vi "LINC Handshake.vi"(7 "GUID (optional)":string, 8 "error in (no error)":errorcluster, 11 "LINC session":refnum<class "LINC.lvclass">) -> (0 "error out":errorcluster, 3 "dup LINC session":refnum<class "LINC.lvclass">)   [LabVIEW 2018, in "STEPkgDriver_LINC.lvlib" / "LINC.lvclass"]
uses:
  LINC.lvclass
  LINC Handshake.ctl
  STEPkgDriver_LINC.lvlib
  LINC Command Origin.ctl
  LINC Global Handshake Mode.ctl
  LINC Handshake Internal.ctl
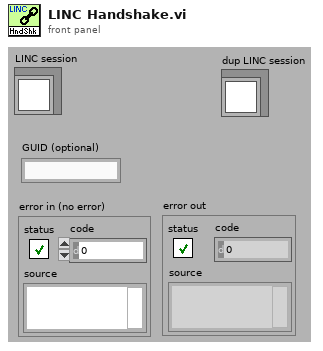
[diagram p1: front panel]
types:
  T1 = typedef "STEPkgDriver_LINC.lvlib/LINC Global Handshake Mode.ctl" = enum16{"INIT", "CLEAR", "ADD_COMMAND", "RMV_COMMAND", "CLR_HANDSHAKE", "SET_HANDSHAKE", "GET_HANDSHAKE"}
  T2 = typedef "STEPkgDriver_LINC.lvlib/LINC Handshake.ctl" = cluster{"ORIGIN":T3, "STATUS":bool, "CODE":i32, "TIME_SECONDS":u32, "TIME_MICROSECONDS":u32, "DATA":string}
  T3 = typedef "STEPkgDriver_LINC.lvlib/LINC Command Origin.ctl" = enum8{"RMT", "LCL"}
  T4 = typedef "STEPkgDriver_LINC.lvlib/LINC Command.ctl" = cluster{"command origin":T3, "command":string, "command data":string}
  T5 = typedef "LVDateTimeRec.ctl" = cluster{"fractional second":dbl, "second":i32, "minute":i32, "hour":i32, "day of month":i32, "month":i32, "year":i32, "day of week":i32, "day of year":i32, "DST":i32}
  T6 = typedef "STEPkgDriver_LINC.lvlib/LINC Handshake Internal.ctl" = cluster{"error":errorcluster, "command data":string}
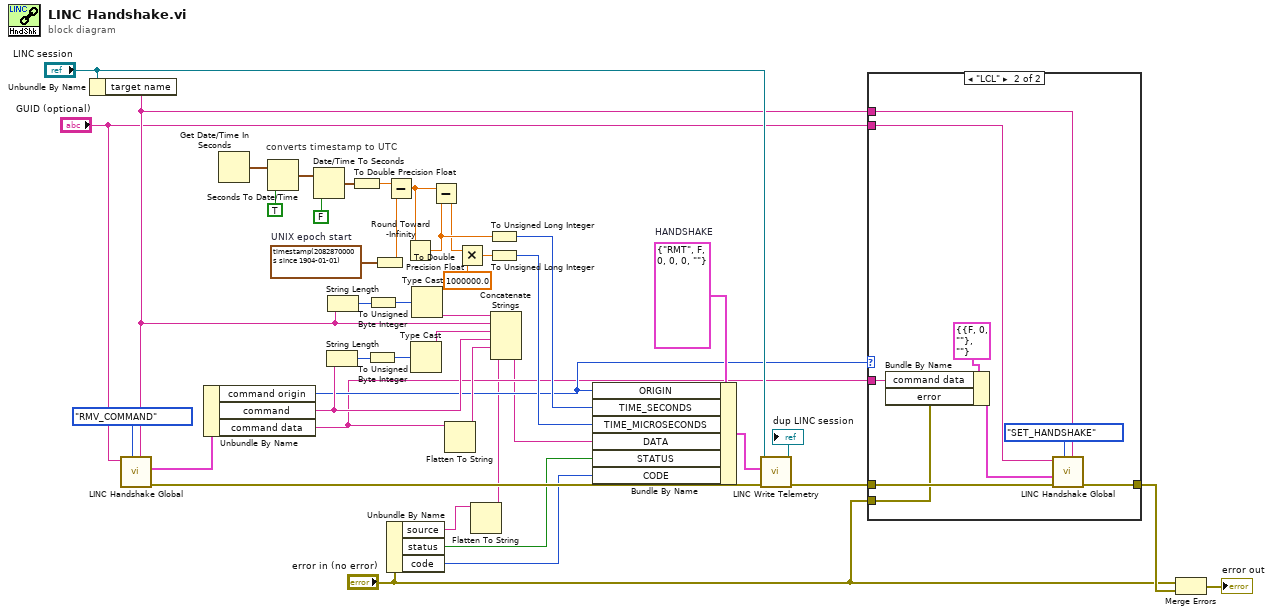
[diagram p0: block diagram]
diagram:
  w29 = timestamp(2082870000 s since 1904-01-01)  # UNIX epoch start
  w32 = T2 {"ORIGIN"=enum."RMT", "STATUS"=FALSE, "CODE"=0, "TIME_SECONDS"=0, "TIME_MICROSECONDS"=0, "DATA"=""}  # HANDSHAKE
  # "converts timestamp to UTC"
  n1 = Unbundle By Name("LINC session") -> ("target name"=w13:string)
  n2 = call "LINC Handshake Global.vi"("target name"=w13, "mode"=LINC_Global_Handshake_Mode."RMV_COMMAND", "GUID"="GUID (optional)") -> ("error out"=w42:errorcluster, "command out"=w9:T4)  [unwired: 5 in, 2 out]
  n3 = Unbundle By Name(w9) -> ("command origin"=w17:T3, "command"=w34:string, "command data"=w7:string)
  n4 = Get Date/Time In Seconds() -> (seconds since 1Jan1904=w8:timestamp)
  n5 = Seconds To Date/Time(time stamp (now)=w8, to UTC (F)=TRUE) -> (date time rec=w19:T5)
  n6 = Date/Time To Seconds(1:FALSE ("is UTC (F)"), 2:w19) -> (0:w18:timestamp)
  n7 = String Length(string=w34) -> (length=w36:i32)
  n8 = String Length(string=w13) -> (length=w40:i32)
  n9 = To Double Precision Float(number=w18) -> (double precision float=w31:dbl)
  n10 = To Unsigned Byte Integer(number=w36) -> (unsigned 8bit integer=w37:u8)
  n11 = To Unsigned Byte Integer(number=w40) -> (unsigned 8bit integer=w39:u8)
  n12 = To Double Precision Float(number=w29) -> (double precision float=w30:dbl)
  n13 = Subtract(x=w31, y=w30) -> (x-y=w28:dbl)
  n14 = Unbundle By Name("error in (no error)") -> ("source"=w3:string, "status"=w5:bool, "code"=w4:i32)
  n15 = Round Toward -Infinity(1:w28) -> (0:w23:dbl)
  n16 = Type Cast(x=w37) -> (*(type *) &x=w35:string)  [unwired: 1 in]
  n17 = Type Cast(x=w39) -> (*(type *) &x=w38:string)  [unwired: 1 in]
  n18 = Subtract(x=w28, y=w23) -> (x-y=w22:dbl)
  n19 = Flatten To String(anything=w7) -> (data string=w33:string)  [unwired: 3 in, 2 out]
  n20 = Multiply(x=w22, y=1000000.0) -> (x*y=w25:dbl)
  n21 = Flatten To String(anything=w3) -> (data string=w2:string)  [unwired: 3 in, 2 out]
  n22 = To Unsigned Long Integer(number=w23) -> (unsigned 32bit integer=w27:u32)
  n23 = To Unsigned Long Integer(number=w25) -> (unsigned 32bit integer=w24:u32)
  n24 = Concatenate Strings(w38, w13, w35, w34, w33, w2) -> (w1:string)
  n25 = Bundle By Name(cluster=w32, "ORIGIN"=w17, "TIME_SECONDS"=w27, "TIME_MICROSECONDS"=w24, "DATA"=w1, "STATUS"=w5, "CODE"=w4) -> (w10:T2)
  n26 = call "LINC Write Telemetry.vi"("error in (no error)"=w42, "packet"=w10, "LINC session"="LINC session") -> ("error out"=w14:errorcluster, "dup LINC session"=→"dup LINC session":refnum<class "LINC.lvclass">)  [unwired: 7 in]
  n27 = case shown="\"LCL\"" w17 {
    tunnel: w14 -> [w44 w52]
    tunnel: [w44 w51] -> w12
    tunnel: w13 -> [_ w50]
    tunnel: "GUID (optional)" -> [_ w49]
    tunnel: w7 -> [_ w47]
    tunnel: "error in (no error)" -> [_ w45]
    frame Default {
    }
    frame "LCL" {
      n28 = Bundle By Name(cluster=T6 {"error"={"status"=FALSE, "code"=0, "source"=""}, "command data"=""} ("handshake"), "command data"=w47, "error"=w45) -> (w46:T6)
      n29 = call "LINC Handshake Global.vi"("target name"=w50, "mode"=LINC_Global_Handshake_Mode."SET_HANDSHAKE", "error in (no error)"=w52, "handshake in"=w46, "GUID"=w49) -> ("error out"=w51:errorcluster)  [unwired: 3 in, 3 out]
    }
  }
  n30 = Merge Errors("error in (no error)", w12) -> (→"error out":errorcluster)
